vi "Get VISA Ref.vi"(8 "error in (no error)":errorcluster, 11 "Temp01 in":refnum<class "TELLC_Temp01.lvclass">) -> (0 "error out":errorcluster, 2 "VISA-placeholder":refnum<visa-resource-name>, 3 "Temp01 out":refnum<class "TELLC_Temp01.lvclass">)   [LabVIEW 2017, in "TELLC_Temp01.lvclass"]
doc: "Developed by Kevin Thompson\nkevin@thompsonengineering.net\n\nCopyright 2018\nThompson Engineering, LLC"
uses:
  TELLC_Temp01.lvclass
  TELLC_Temp01.lvclass/TELLC_Temp01.ctl
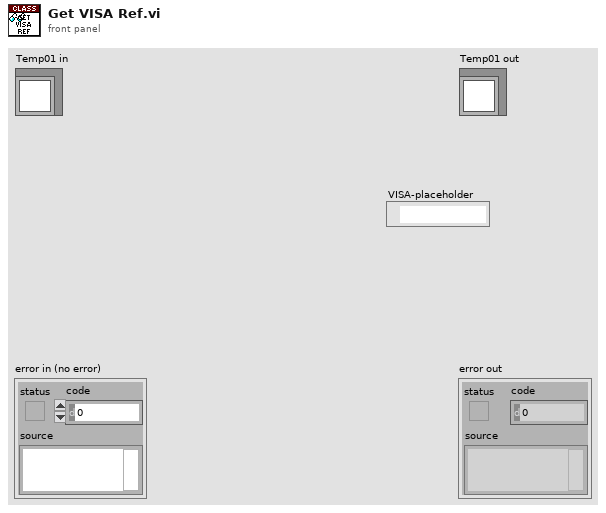
[diagram p1: front panel]
types:
  T1 = typedef "TELLC_Temp01.lvclass/ObjData--cluster.ctl" = cluster{"Settings":T2, "ReadData-placeholder":T3, "VISA-placeholder":refnum<visa-resource-name>}
  T2 = typedef "TELLC_Temp01.lvclass/Settings--cluster.ctl" = cluster{"Simulation":bool}
  T3 = typedef "TELLC_Temp01.lvclass/Read Data--cluster.ctl" = cluster{"Data":dbl}
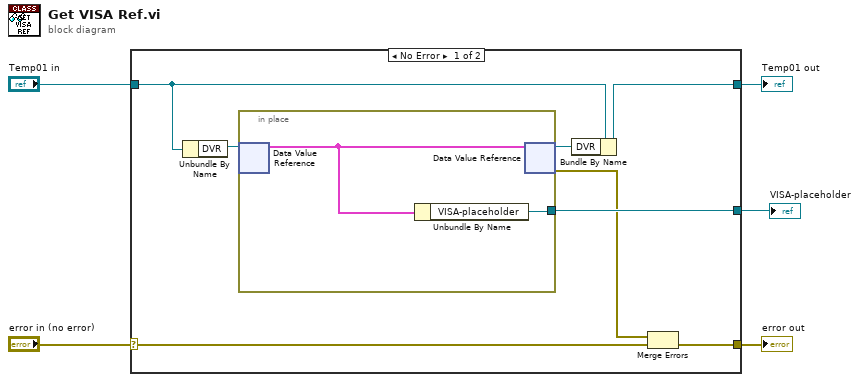
[diagram p0: block diagram]
diagram:
  n1 = case shown="No Error" "error in (no error)" {
    selector: "error in (no error)" -> [w13 w16]
    tunnel: [w7 w16] -> w4
    tunnel: [w9 w17] -> w2
    tunnel: "Temp01 in" -> [w10 w17]
    tunnel: [w8 _] -> w1
    frame No Error {
      n2 = Unbundle By Name(w10) -> ("DVR"=w11:refnum<data-value>)
      n3 = in-place {
        in-place-border: [w14] -> w8
        n4 = in-place-dvr #1(w11) -> (w15:T1)  [unwired: 1 out]
        n5 = Unbundle By Name(w15) -> ("VISA-placeholder"=w14:refnum<visa-resource-name>)
        n6 = in-place-dvr #1(w15) -> (w12:refnum<data-value>, w6:errorcluster)
      }
      n7 = Bundle By Name(cluster=w10, "DVR"=w12) -> (w9:refnum<class "TELLC_Temp01.lvclass">)
      n8 = Merge Errors(w6, w13) -> (w7:errorcluster)
    }
    frame Error {
    }
  }
  "error out" <- w4
  "Temp01 out" <- w2
  "VISA-placeholder" <- w1
